vi "RADIX2DIT.vi"() -> ()   [LabVIEW 2014]
uses:
  <vilib>/Analysis/2dsp.llb/Real FFT.vi
  <vilib>/Analysis/NI_AALPro.lvlib
panel:
  in  "stop":bool
  out "Waveform Chart 2":dbl[](graph)
  in  "INPUT":dbl[](array[numeric])
  out "Waveform Chart":dbl[](graph)
  out "FFT {X}":cdb[](array[numeric]) format="%#.3f"
  out "FORMULA'S OUTPUT":cdb[](array[numeric]) format="%#.3f"
  in  "N":dbl
  # "RADIX-2 DIT FFT"
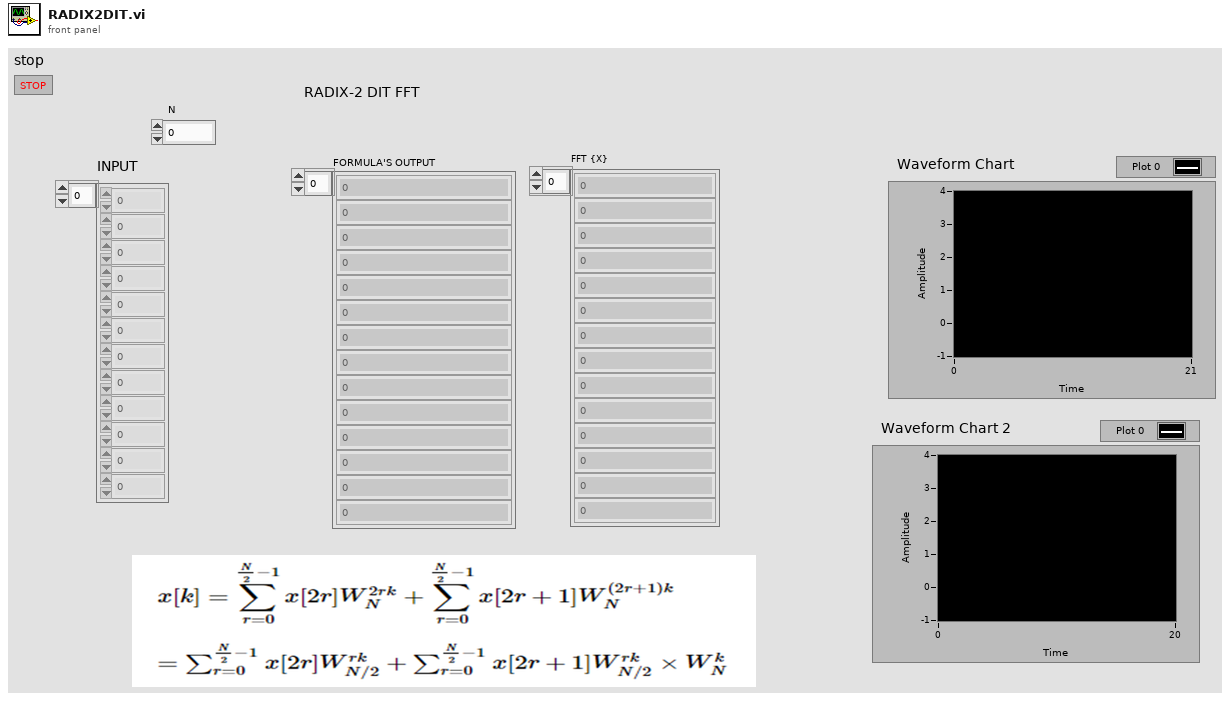
[diagram p1: front panel]
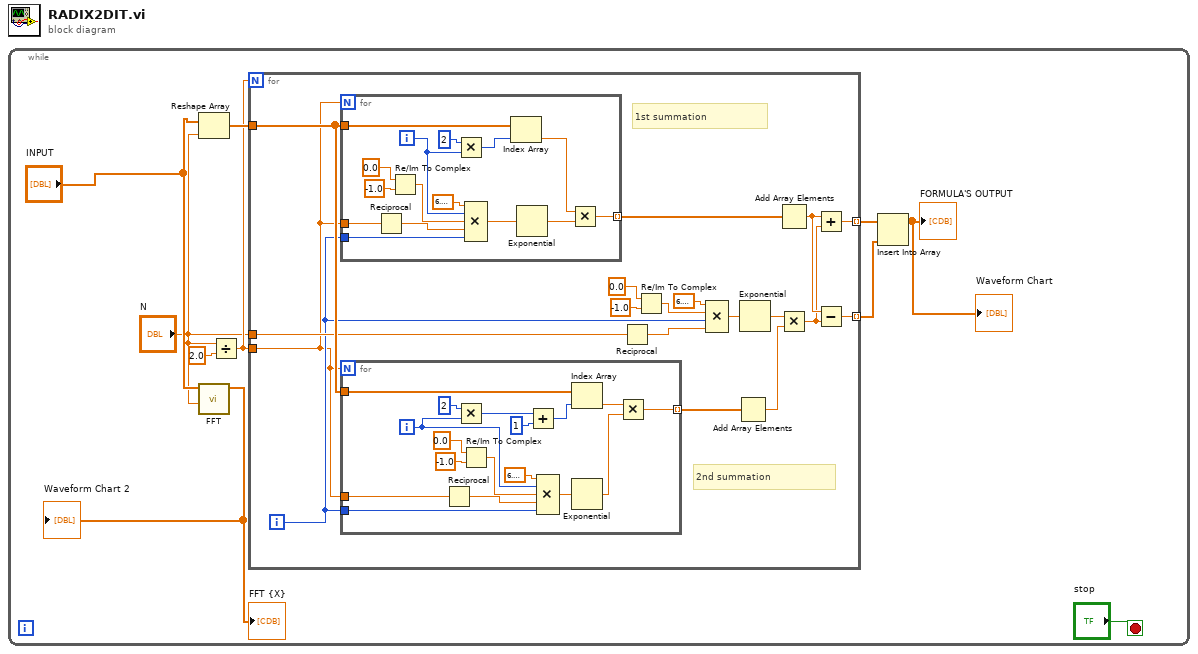
[diagram p0: block diagram]
diagram:
  n1 = while {
    stop <- "stop" stop-if-true
    n2 = Reshape Array("INPUT", "N") -> (w10:dbl[])
    n3 = call-poly <vilib>:"FFT.vi"("FFT size"="N", "X"="INPUT") -> ("FFT {X}"=→"FFT {X}" →"Waveform Chart 2":cdb[])  [unwired: 8 in, 1 out]
    n4 = Divide(x="N", y=2.0) -> (x/y=w7:dbl)
    n5 = for {
      N: w7 -> [_]
      tunnel: w10 -> [w22]
      tunnel: "N" -> [w21]
      tunnel: w7 -> [w15]
      tunnel: [w12] -> w8 mode=indexing
      tunnel: [w11] -> w6 mode=indexing
      i -> [w18]
      # "2nd summation"
      # "1st summation"
      n6 = for {
        N: w15 -> [_]
        tunnel: w22 -> [w58]
        tunnel: w15 -> [w47]
        tunnel: [w49] -> w28 mode=indexing
        tunnel: w18 -> [w48]
        i -> [w53]
        n7 = Reciprocal(x=w47) -> (1/x=w46:dbl)
        n8 = Re/Im To Complex(1:-1.0 ("y"), 2:0.0 ("x")) -> (0:w54:cdb)
        n9 = Multiply(x=2, y=w53) -> (x*y=w59:i32)
        n10 = Compound Arithmetic op=MULTIPLY(6.283185307179586, w53, w54, w46, w48) -> (w52:cdb)
        n11 = Index Array(array=w58, index=w59) -> (element=w51:dbl)
        n12 = Exponential(1:w52) -> (0:w50:cdb)
        n13 = Multiply(x=w51, y=w50) -> (x*y=w49:cdb)
      }
      n14 = for {
        N: w15 -> [_]
        tunnel: w22 -> [w43]
        tunnel: w15 -> [w30]
        tunnel: [w34] -> w27 mode=indexing
        tunnel: w18 -> [w31]
        i -> [w38]
        n15 = Reciprocal(x=w30) -> (1/x=w29:dbl)
        n16 = Multiply(x=2, y=w38) -> (x*y=w44:i32)
        n17 = Re/Im To Complex(1:-1.0 ("y"), 2:0.0 ("x")) -> (0:w39:cdb)
        n18 = Add(x=w44, y=1) -> (x+y=w33:i32)
        n19 = Compound Arithmetic op=MULTIPLY(6.283185307179586, w38, w39, w29, w31) -> (w37:cdb)
        n20 = Index Array(array=w43, index=w33) -> (element=w36:dbl)
        n21 = Exponential(1:w37) -> (0:w35:cdb)
        n22 = Multiply(x=w36, y=w35) -> (x*y=w34:cdb)
      }
      n23 = Reciprocal(x=w21) -> (1/x=w20:dbl)
      n24 = Re/Im To Complex(1:-1.0 ("y"), 2:0.0 ("x")) -> (0:w23:cdb)
      n25 = Compound Arithmetic op=MULTIPLY(6.283185307179586, w23, w18, w20) -> (w19:cdb)
      n26 = Add Array Elements(numeric array=w27) -> (sum=w16:cdb)
      n27 = Exponential(1:w19) -> (0:w17:cdb)
      n28 = Add Array Elements(numeric array=w28) -> (sum=w14:cdb)
      n29 = Multiply(x=w17, y=w16) -> (x*y=w13:cdb)
      n30 = Add(x=w14, y=w13) -> (x+y=w12:cdb)
      n31 = Subtract(x=w14, y=w13) -> (x-y=w11:cdb)
    }
    n32 = Insert Into Array(array=w8, new element=w6) -> (→"FORMULA'S OUTPUT" →"Waveform Chart":cdb[])  [unwired: 1 in]
  }
